vi "压力数据保存判定 - 夹爪.vi"(7 "路径":path, 9 "布尔":bool, 11 "添加的数组":dbl[](array[numeric])) -> ()   [LabVIEW 2017]
uses:
  <vilib>/Utility/file.llb/Write Delimited Spreadsheet (string).vi
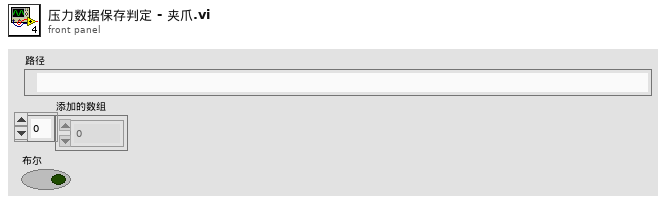
[diagram p1: front panel]
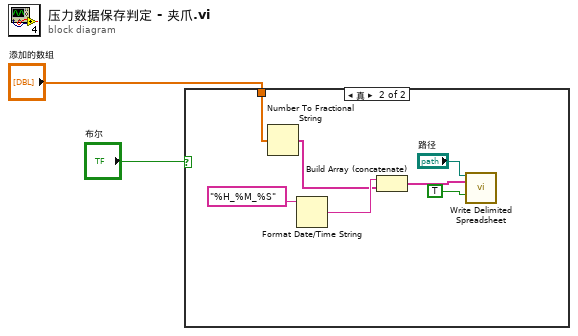
[diagram p0: block diagram]
diagram:
  n1 = case shown="真" "布尔" {
    tunnel: "添加的数组" -> [_ w6]
    frame False {
    }
    frame True {
      n2 = Number To Fractional String(number=w6) -> (F-format string=w5:string[])  [unwired: 3 in]
      n3 = Format Date/Time String(time format string (%c)="%H_%M_%S" ("时间格式字符串(%c)")) -> (date/time string=w7:string)  [unwired: 2 in]
      n4 = Build Array (concatenate)(w7, w5) -> (w4:string[])
      n5 = call-poly <vilib>:"Write Delimited Spreadsheet.vi"("file path (dialog if empty)"="路径", "1D data"=w4, "append to file? (new file:F)"=TRUE) -> ()  [unwired: 11 in, 2 out]
    }
  }
